vi "Untitled 1.vi"() -> ()   [LabVIEW 2019, in "Computer_SVs.lvlib"]
uses:
  Computer_SVs.lvlib
panel:
  out "?":dbl
  out "wh":dbl
  # "rl"
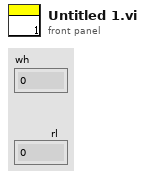
[diagram p1: front panel]
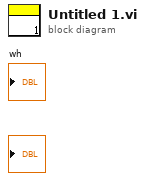
[diagram p0: block diagram]
diagram:
